vi "Log Control Event.vi"(8 "error in (no error)":errorcluster, 11 "Control In":refnum<vi>) -> (0 "error out":errorcluster)   [LabVIEW 2020]
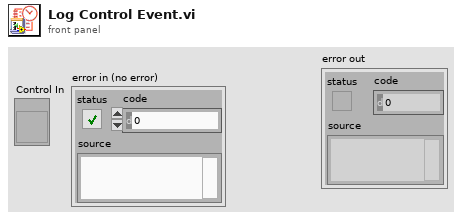
[diagram p1: front panel]
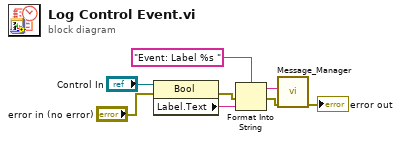
[diagram p0: block diagram]
diagram:
  n1 = property class="Bool"(reference="Control In", error in="error in (no error)") -> (error out=w4:errorcluster, "Label.Text"=w7:string)  [unwired: 1 out]
  n2 = Format Into String(format string="Event: Label %s " ("New Entry"), error in=w4, w7) -> (resulting string=w8:string, error out=w3:errorcluster)  [unwired: 1 in]
  n3 = call "Message_Manager.vi"("error in"=w3, "New Entry"=w8) -> ("error out"=→"error out":errorcluster)  [unwired: 5 in, 4 out]
